vi "GetLimits.vi"(8 "error in (no error)":errorcluster, 10 "Axis":T1 items=["1"=1, "2"=2, "3"=3, "4"=4], 11 "DelayLineSimulation in":refnum<class "DelayLineSimulation.lvclass">) -> (0 "error out":errorcluster, 1 "max":dbl, 2 "min":dbl, 3 "DelayLineSimulation out":refnum<class "DelayLineSimulation.lvclass">)   [LabVIEW 2015]
uses:
  DelayLineLS4/LS4 axis.ctl
  DelayLine.lvclass
  DelayLineSimulation.lvclass
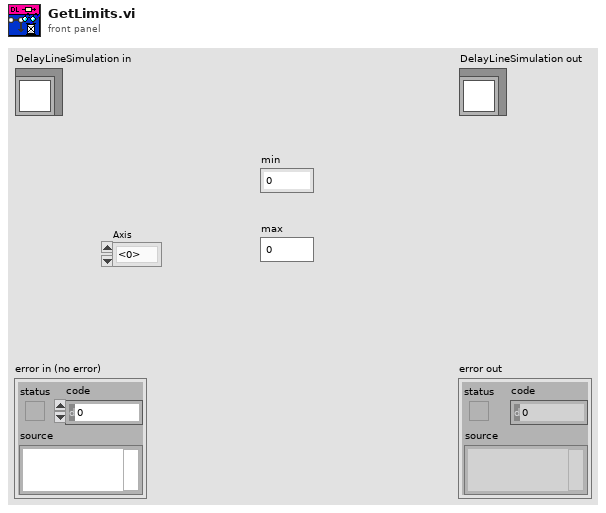
[diagram p1: front panel]
types:
  T1 = typedef "DelayLine.lvclass/LS4 axis.ctl" = u16
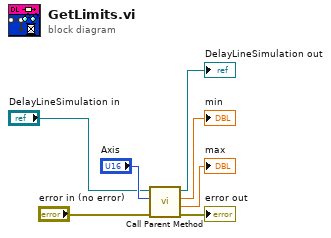
[diagram p0: block diagram]
diagram:
  n1 = call-parent "Call Parent Method"("error in (no error)"="error in (no error)", "Axis"="Axis", "DelayLine in"="DelayLineSimulation in") -> ("error out"=→"error out":errorcluster, "max"=→"max":dbl, "min"=→"min":dbl, "DelayLine out"=→"DelayLineSimulation out":refnum<class "DelayLineSimulation.lvclass">)  [unwired: 5 in]
